vi "Write ENET Init Settings.vi"(5 "Auto-Refresh (T)":bool=TRUE, 6 "UDP port":u16=54321, 7 "Connect for Config Only? (F)":bool, 8 "error in (no error)":errorcluster, 9 "TCP port":u16=12345, 10 "Box IP address":string="192.168.1.100", 11 "Ethernet_BS1201 in":refnum<class "ENET_BS120x.lvclass">) -> (0 "error out":errorcluster, 3 "Ethernet_BS1201 out":refnum<class "ENET_BS120x.lvclass">)   [LabVIEW 2021, in "BS120x Driver.lvlib" / "ENET_BS120x.lvclass"]
uses:
  ENET_BS120x.lvclass
  ENET_BS120x.lvclass/ENET_BS120x.ctl
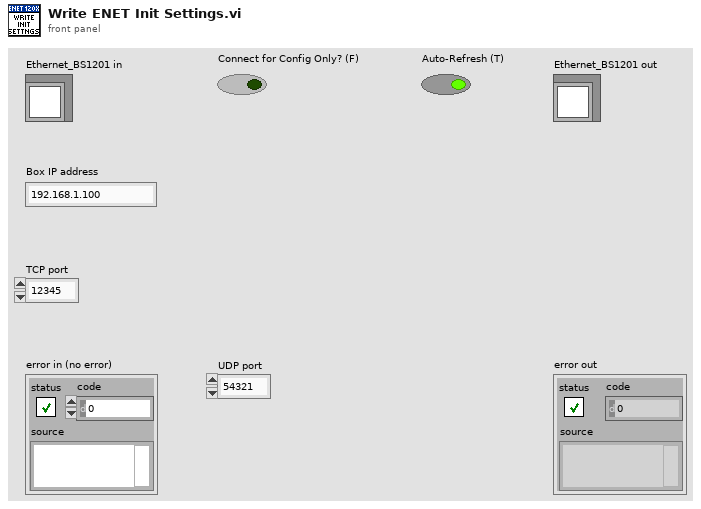
[diagram p1: front panel]
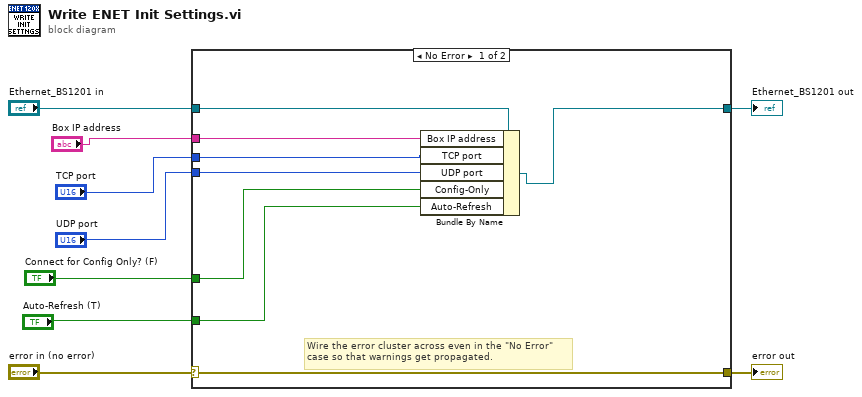
[diagram p0: block diagram]
diagram:
  n1 = case shown="No Error" "error in (no error)" {
    selector: "error in (no error)" -> [w17 w19]
    tunnel: [w17 w19] -> w8
    tunnel: [w10 w18] -> w6
    tunnel: "Ethernet_BS1201 in" -> [w16 w18]
    tunnel: "Box IP address" -> [w15 _]
    tunnel: "TCP port" -> [w14 _]
    tunnel: "UDP port" -> [w13 _]
    tunnel: "Connect for Config Only? (F)" -> [w12 _]
    tunnel: "Auto-Refresh (T)" -> [w11 _]
    frame No Error {
      # "Wire the error cluster across even in the \"No Error\"\ncase so that warnings get propagated."
      n2 = Bundle By Name(cluster=w16, "Box IP address"=w15, "TCP port"=w14, "UDP port"=w13, "Config-Only"=w12, "Auto-Refresh"=w11) -> (w10:refnum<class "ENET_BS120x.lvclass">)
    }
    frame Error {
    }
  }
  "error out" <- w8
  "Ethernet_BS1201 out" <- w6
